vi "prepAOWaveplot.vi"(1 "WaveformGraph in":refnum<vi>, 2 "Analog Used Names":string[](array[string])) -> ()   [LabVIEW 2015]
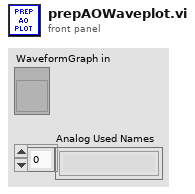
[diagram p1: front panel]
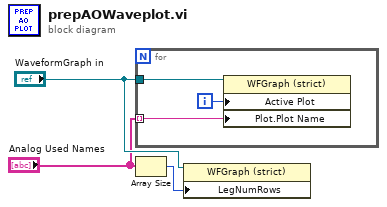
[diagram p0: block diagram]
diagram:
  n1 = for {
    tunnel: "WaveformGraph in" -> [w6]
    tunnel: "Analog Used Names" -> [w5] mode=indexing
    i -> [w4]
    n2 = property on="Property Node" class="WFGraph (strict)"(reference=w6, "Active Plot"=w4, "Plot.Plot Name"=w5) -> ()  [unwired: 1 in, 2 out]
  }
  n3 = Array Size(array="Analog Used Names") -> (size(s)=w3:i32)
  n4 = property on="Property Node" class="WFGraph (strict)"(reference="WaveformGraph in", "LegNumRows"=w3) -> ()  [unwired: 1 in, 2 out]
